vi "Directory.vi"() -> (1 "Directory":path)   [LabVIEW 2019]
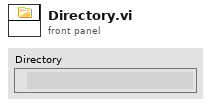
[diagram p1: front panel]
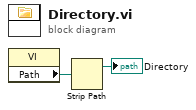
[diagram p0: block diagram]
diagram:
  n1 = property class="VI"() -> ("Path"=w1:path)  [unwired: 2 in, 2 out]
  n2 = Strip Path(path=w1) -> (stripped path=→"Directory":path)  [unwired: 1 out]
